vi "CallInputList.vi"(5 "list":string, 9 "SubVI in":refnum<class "SubVI.lvclass">) -> (3 "SubVI out":refnum<class "SubVI.lvclass">, 4 "call inputs":string[](array[string]))   [LabVIEW 2014, in "Raspberry Pi Compatible Compiler for LabVIEW.lvlib" / "SubVI.lvclass"]
uses:
  SubVI.lvclass
  Node/Node.lvclass
  Terminal/Terminal.lvclass
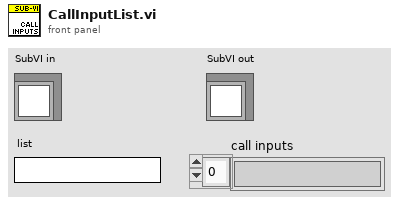
[diagram p1: front panel]
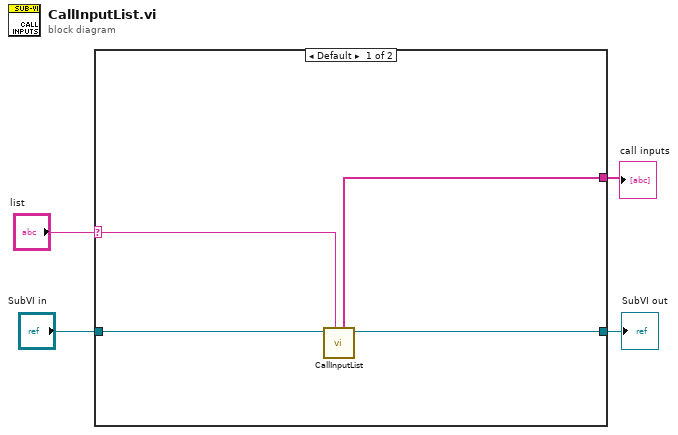
[diagram p0: block diagram]
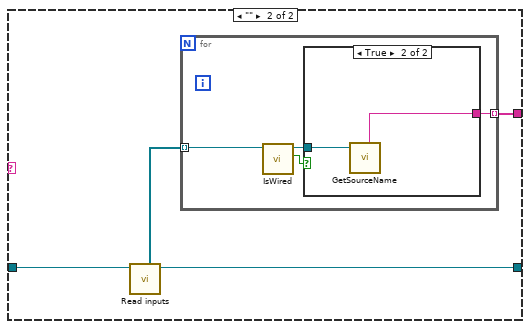
[diagram p2: hidden frame]
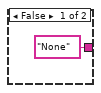
[diagram p3: hidden frame]
diagram:
  n1 = case shown="Default" "list" {
    selector: "list" -> [w7 _]
    tunnel: "SubVI in" -> [w8 w11]
    tunnel: [w6 w10] -> w3
    tunnel: [w5 w9] -> w2
    frame Default {
      n2 = call-parent "CallInputList.vi"("list"=w7, "Node in"=w8) -> ("Node out"=w5:refnum<class "SubVI.lvclass">, "call inputs"=w6:string[])  [unwired: 6 in]
    }
    frame "" {
      n3 = call-dynamic "Read inputs.vi"("Node in"=w11) -> ("Node out"=w9:refnum<class "SubVI.lvclass">, "inputs"=w12:refnum<class "Terminal.lvclass">[])  [unwired: 7 in]
      n4 = for {
        tunnel: w12 -> [w13] mode=indexing
        tunnel: [w16] -> w10 mode=indexing
        n5 = call "IsWired.vi"("Terminal in"=w13) -> ("wired"=w14:bool, "Terminal out"=w15:refnum<class "Terminal.lvclass">)  [unwired: 6 in, 1 out]
        n6 = case shown="True" w14 {
          tunnel: ["None" w18] -> w16
          tunnel: w15 -> [_ w19]
          frame False {
          }
          frame True {
            n7 = call "GetSourceName.vi"("Terminal in"=w19) -> ("source"=w18:string)  [unwired: 6 in, 2 out]
          }
        }
      }
    }
  }
  "SubVI out" <- w2
  "call inputs" <- w3
